vi "Call gRPC Scripting.vi"(8 "error in":errorcluster, 10 "Proto Names":T1, 11 "proto File Path":path) -> (0 "error out":errorcluster)   [LabVIEW 2021, in "Plugin Generator.lvlib"]
uses:
  Plugin Generator.lvlib
  Typedef/Proto Names.ctl
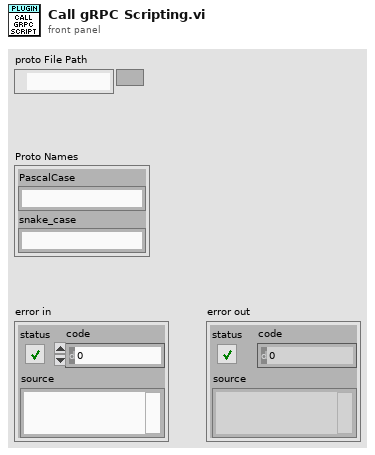
[diagram p1: front panel]
types:
  T1 = typedef "Plugin Generator.lvlib/Proto Names.ctl" = cluster{"PascalCase":string, "snake_case":string}
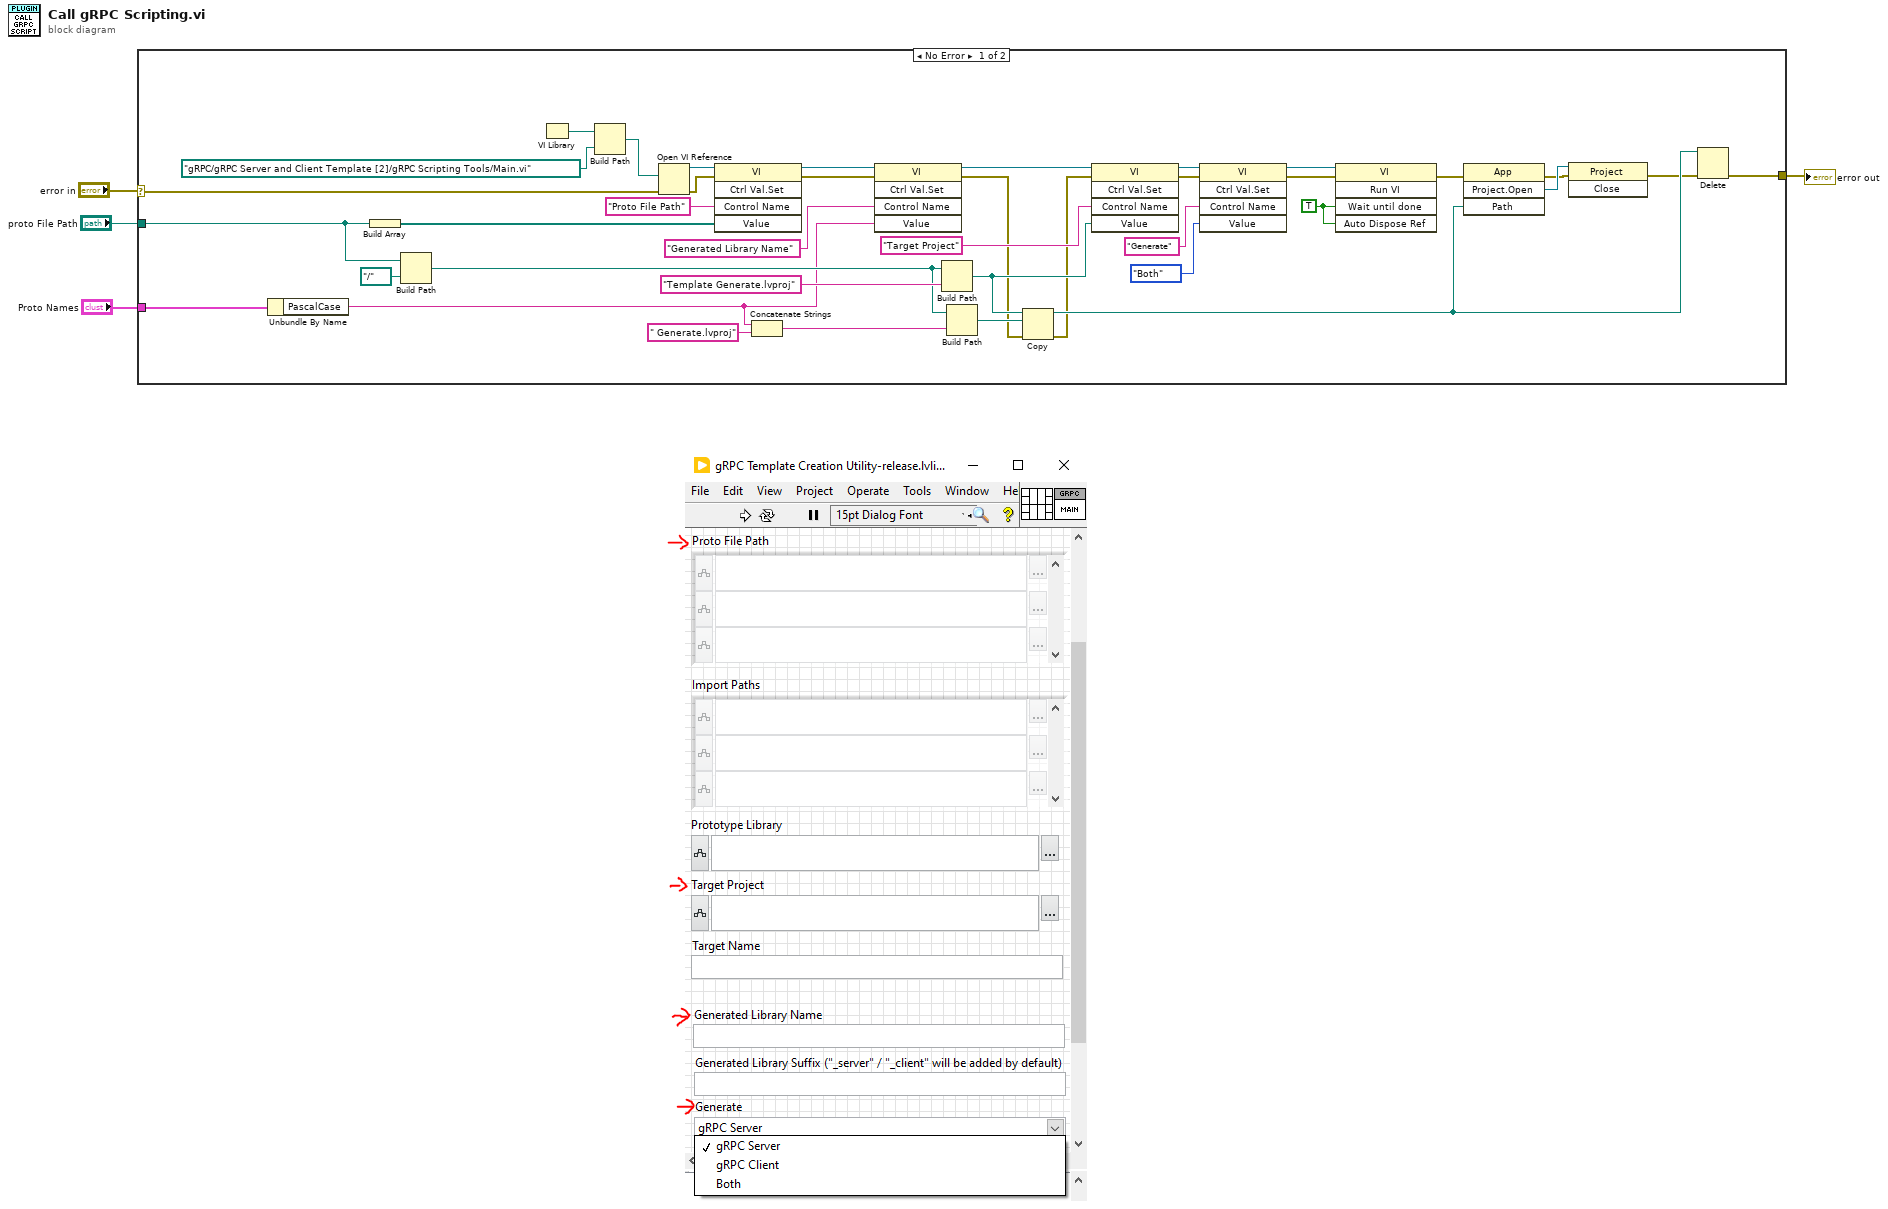
[diagram p0: block diagram]
diagram:
  n1 = case shown="No Error" "error in" {
    selector: "error in" -> [w7 w42]
    tunnel: [w12 w42] -> w4
    tunnel: "proto File Path" -> [w18 _]
    tunnel: "Proto Names" -> [w5 _]
    frame No Error {
      w19 = TRUE ("Wait Until Done")
      n2 = Unbundle By Name(w5) -> ("PascalCase"=w6:string)
      n3 = Build Array(w18) -> (w24:path[])
      n4 = Build Path(base path=w18, name or relative path=path "../..") -> (appended path=w15:path)
      n5 = VI Library() -> (path=w41:path)
      n6 = Build Path(base path=w41, name or relative path=path "gRPC/gRPC Server and Client Template [2]/gRPC Scripting Tools/Main.vi") -> (appended path=w39:path)
      n7 = Open VI Reference(vi path=w39, error in (no error)=w7) -> (vi reference=w26:refnum<vi>, error out=w25:errorcluster)  [unwired: 4 in]
      n8 = invoke class="VI" method="Ctrl Val.Set"(reference=w26, error in=w25, "Control Name"="Proto File Path", "Value"=w24) -> (reference out=w37:refnum<vi>, error out=w36:errorcluster)  [unwired: 1 in, 3 out]
      n9 = Concatenate Strings(w6, " Generate.lvproj" ("string")) -> (w14:string)
      n10 = invoke class="VI" method="Ctrl Val.Set"(reference=w37, error in=w36, "Control Name"="Generated Library Name", "Value"=w6) -> (reference out=w34:refnum<vi>, error out=w10:errorcluster)  [unwired: 1 in, 3 out]
      n11 = Build Path(base path=w15, name or relative path="Template Generate.lvproj" ("string")) -> (appended path=w11:path)
      n12 = Build Path(base path=w15, name or relative path=w14) -> (appended path=w13:path)
      n13 = Copy(8:w10, 10:w13, 11:w11) -> (0:w9:errorcluster)  [unwired: 2 in, 2 out]
      n14 = invoke class="VI" method="Ctrl Val.Set"(reference=w34, error in=w9, "Control Name"="Target Project", "Value"=w11) -> (reference out=w32:refnum<vi>, error out=w31:errorcluster)  [unwired: 1 in, 3 out]
      n15 = invoke class="VI" method="Ctrl Val.Set"(reference=w32, error in=w31, "Control Name"="Generate", "Value"=enum16{"gRPC Server", "gRPC Client", "Both"}."Both" ("Generate")) -> (reference out=w28:refnum<vi>, error out=w27:errorcluster)  [unwired: 1 in, 3 out]
      n16 = invoke class="VI" method="Run VI"(reference=w28, error in=w27, "Wait until done"=w19, "Auto Dispose Ref"=w19) -> (error out=w20:errorcluster)  [unwired: 1 in, 4 out]
      n17 = invoke class="App" method="Project.Open"(error in=w20, "Path"=w11) -> (error out=w21:errorcluster, "Project:Open"=w22:refnum<vi>)  [unwired: 2 in, 2 out]
      n18 = invoke class="Project" method="Close"(reference=w22, error in=w21) -> (error out=w8:errorcluster)  [unwired: 1 in, 2 out]
      n19 = Delete(path (use dialog)=w11, error in=w8) -> (error out=w12:errorcluster)  [unwired: 3 in, 2 out]
    }
    frame Error {
    }
  }
  "error out" <- w4
